vi "Get Image.vi"(8 "error in (no error)":errorcluster, 11 "Simulated in":refnum<class "Simulated Camera.lvclass">) -> (0 "error out":errorcluster, 2 "Image":u16[][](array[numeric]), 3 "Simulated out":refnum<class "Simulated Camera.lvclass">)   [LabVIEW 2019, in "Simulated Camera.lvclass"]
uses:
  Simulated Camera.lvclass
  Simulated Camera.lvclass/Simulated Camera.ctl
  <vilib>/numeric/Random Number (Range) U64.vi
  <vilib>/numeric/sub_Random U32.vi
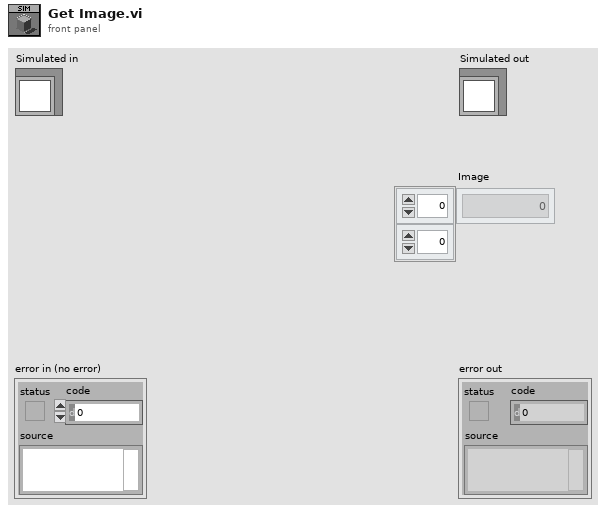
[diagram p1: front panel]
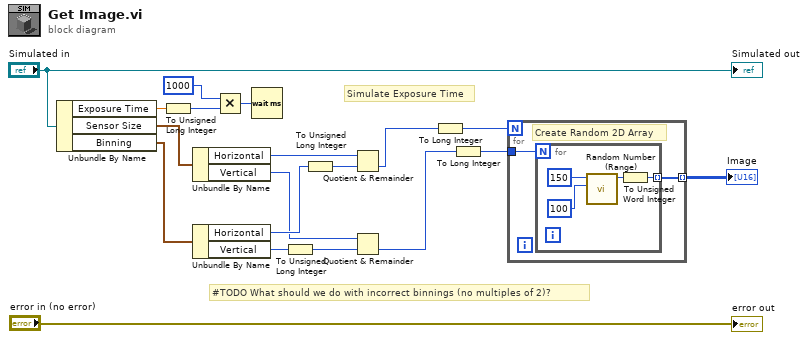
[diagram p0: block diagram]
diagram:
  # "#TODO What should we do with incorrect binnings (no multiples of 2)?"
  # "Simulate Exposure Time"
  n1 = Unbundle By Name("Simulated in") -> ("Exposure Time"=w16:dbl, "Sensor Size"=w11:cluster{"Horizontal":u32, "Vertical":u32}, "Binning"=w12:cluster{"Horizontal":u16, "Vertical":u16})
  n2 = To Unsigned Long Integer(number=w16) -> (unsigned 32bit integer=w15:u32)
  n3 = Unbundle By Name(w11) -> ("Horizontal"=w10:u32, "Vertical"=w7:u32)
  n4 = Unbundle By Name(w12) -> ("Horizontal"=w9:u16, "Vertical"=w6:u16)
  n5 = Multiply(x=u32 1000, y=w15) -> (x*y=w14:u32)
  n6 = Wait (ms)(milliseconds to wait=w14) -> ()  [unwired: 1 out]
  n7 = To Unsigned Long Integer(number=w6) -> (unsigned 32bit integer=w5:u32)
  n8 = To Unsigned Long Integer(number=w9) -> (unsigned 32bit integer=w8:u32)
  n9 = Quotient & Remainder(x=w10, y=w8) -> (floor(x/y)=w4:u32)  [unwired: 1 out]
  n10 = Quotient & Remainder(x=w7, y=w5) -> (floor(x/y)=w3:u32)  [unwired: 1 out]
  n11 = To Long Integer(number=w4) -> (32bit integer=w2:i32)
  n12 = To Long Integer(number=w3) -> (32bit integer=w1:i32)
  n13 = for {
    N: w2 -> [_]
    tunnel: [w21] -> w19 mode=indexing
    tunnel: w1 -> [w20]
    # "Create Random 2D Array"
    n14 = for {
      N: w20 -> [_]
      tunnel: [w24] -> w21 mode=indexing
      n15 = call-poly <vilib>:"Random Number (Range).vi"("lower bound (0)"=u64 100, "upper bound (100)"=u64 150) -> ("number"=w25:u64)  [unwired: 9 in]
      n16 = To Unsigned Word Integer(number=w25) -> (unsigned 16bit integer=w24:u16)
    }
  }
  "Image" <- w19
  "error out" <- "error in (no error)"
  "Simulated out" <- "Simulated in"
